vi "Get Number.vi"(8 "error in (no error)":errorcluster, 11 "Callback Consumer in":refnum<class "Callback Consumer.lvclass">) -> (0 "error out":errorcluster, 2 "Numeric":dbl, 3 "Callback Consumer out":refnum<class "Callback Consumer.lvclass">)   [LabVIEW 2020, in "Callback Consumer.lvclass"]
uses:
  Callback Consumer.lvclass
  Callback Consumer.lvclass/Callback Consumer.ctl
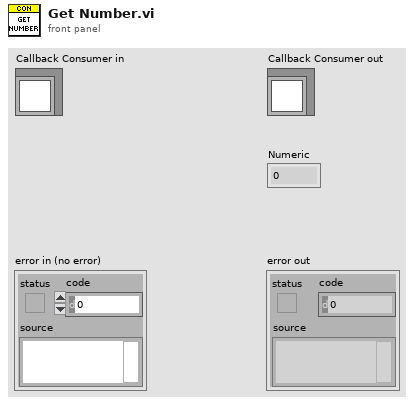
[diagram p1: front panel]
types:
  T1 = typedef "Callback Consumer.lvclass/Ref Data.ctl" = cluster{"Numeric":dbl}
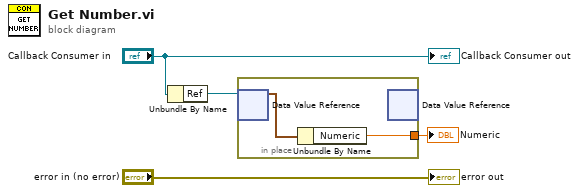
[diagram p0: block diagram]
diagram:
  n1 = Unbundle By Name("Callback Consumer in") -> ("Ref"=w3:refnum<data-value>)
  n2 = in-place {
    in-place-border: [w5] -> w1
    n3 = in-place-dvr #1(w3) -> (w6:T1)  [unwired: 1 out]
    n4 = Unbundle By Name(w6) -> ("Numeric"=w5:dbl)
    n5 = in-place-dvr #1() -> ()  [unwired: 1 in, 2 out]
  }
  "Numeric" <- w1
  "error out" <- "error in (no error)"
  "Callback Consumer out" <- "Callback Consumer in"
